vi "Multi-Device_Sync-AI_and_AO-Shared_Timebase_&_Trig-DSA.vi"() -> ()   [LabVIEW 2013]
doc: "I. Description:\nThis example configures a total of four tasks on two PXI Dynamic Signal Acquistion (DSA) devices. Each device runs a task for analog input and another for analog output. This VI illustrates continuous analog input and ouptut operations.\n\nII. Instructions for Running:\n1. Select which type of Syncrhonization method you want to use.\n2. Select the physical channels to corresponding to the signal connection on each device.\n3. Enter the minimum and maximum expected voltage for the input and output operations on each device.\nNote: For optimal accuracy, match the input range to the expected voltage level of the measured signal (for input) and generated signal (for output).\n4. Set the number of samples to acquire per channel. This parameter determines how many points will be read and generated with each iteration of the WHILE loop.\n5. Set the rate of the acquisition and generation. The same sampling rate is employed for input and output operations on each device.\nNote: The sampling rate should be at least 2.2 times the maximum frequency component of the signal being acquired on analog input and the signal being generated on analog output. Frequency components beyond about 0.47 times the sampling rate will be eliminated by the alias and imaging protection on the DSA device.\n\nIII. Block Diagram Steps:\n1. Create an analog input and output channel for both the master and slave devices.\n2. Set timing parameters for a continuous acquisition. The sample rate and block size are set to the same values for each device.\n3. There are two types of synchronization available on DSA devices. The first method shares the Sample Clock Timebase across the PXI_Star bus. It also uses the Sync Pulse which is shared across the PXI_Trig / RTSI bus. The second method uses the Sync Pulse in conjunction with the PXI Reference clock 10 on the PXI backplane. \n4. Call the Get Terminal Name with Device Prefix VI to append the device name to the signal name for the acquisition start trigger. This signal is then used as an output generation trigger on the master as well as and acquisition start trigger and generation start trigger on the slave. The signal is shared along the PXI_Trig / RTSI bus.\n5. Synthesize a standard waveform (sine, square, or triangle) and load this data into the output RAM buffer for each device.\n6. Call the Start VI to start the acquisition and generation tasks. (Note: The flat case structure provides flow control so that the slave device is armed before the master so that the slave device does not miss the trigger.)\n7. Read all of the waveform data from both devices.\n8. Check the status of the analog output tasks on both devices.\n9. Call the Clear Task VI to stop the acquisition and generation and clear the task.\n10. Use the popup dialog box to display an error if any.\n\nIV. I/O Connections Overview:\nMake sure your signal input and output terminals matches the Physical Channel I/O controls.\n\nIt is important to ensure that your PXI chassis has been properly configured in MAX. If your chassis has not been configured in software before running the VI, your devices may fail to synchronize properly."
uses:
  <vilib>/Utility/error.llb/DialogType.ctl
  <vilib>/DAQmx/write.llb/DAQmx Write (Analog Wfm 1Chan NSamp).vi
  <vilib>/DAQmx/read.llb/DAQmx Read (Analog 1D Wfm NChan NSamp).vi
  <vilib>/DAQmx/create/channels.llb/DAQmx Create Channel (AI-Voltage-Basic).vi
  <vilib>/DAQmx/create/channels.llb/DAQmx Create Channel (AO-Voltage-Basic).vi
  <vilib>/DAQmx/configure/timing.llb/DAQmx Timing (Sample Clock).vi
  <vilib>/DAQmx/configure/trigger.llb/DAQmx Start Trigger (Digital Edge).vi
  <vilib>/DAQmx/miscellaneous.llb/DAQmx Fill In Error Info.vi
  <resource>/objmgr/daqmx.rc
panel:
  in  "Synchronization Type":u16(ring) items=["DSA Sample Clock Timebase", "DSA Reference Clock"]
  out "Resulting Sample \nClock Rate [S/s]":dbl format="%.2f"
  in  "Desired Frequency":dbl=1000.0 format="%.2f"
  in  "Cycles per Buffer":dbl=5.0 format="%.2f"
  in  "Waveform Type":T1(ring)
  in  "Samples per Buffer":dbl=250.0
  in  "Amplitude":dbl=1.0 format="%0.2p"
  in  "Minimum Value":dbl=-10.0 caption="Output Minimum Value" format="%0.2f"
  in  "Maximum Value":dbl=10.0 caption="Output Maximum Value" format="%0.2f"
  in  "Physical Channel":tag="PXI1Slot3/ao0" caption="Slave Output Physical Channels"
  in  "Maximum Value":dbl=10.0 caption="Input Maximum Value" format="%0.2f"
  in  "Minimum Value":dbl=-10.0 caption="Input Minimum Value" format="%0.2f"
  in  "Physical Channel":tag="PXI1Slot3/ai0" caption="Slave Input Physical Channel"
  out "Measurement":waveform(dbl)[](graph) caption="Measurement:  Slave Board"
  in  "Samples per Channel":i32=2000 caption="Samples to Read per Loop"
  in  "Minimum Value":dbl=-10.0 caption="Output Minimum Value" format="%0.2f"
  in  "Maximum Value":dbl=10.0 caption="Output Maximum Value" format="%0.2f"
  in  "Physical Channel":tag="PXI1Slot2/ao0" caption="Master Output Physical Channels"
  in  "Maximum Value":dbl=10.0 caption="Input Maximum Value" format="%0.2f"
  in  "Minimum Value":dbl=-10.0 caption="Input Minimum Value" format="%0.2f"
  in  "Physical Channel":tag="PXI1Slot2/ai0" caption="Master Input Physical Channel"
  in  "stop":bool
  out "Measurement":waveform(dbl)[](graph) caption="Measurement:  Master Board"
  # "For instructions, select Help>>Show Context Help"
  # "Channel Parameters:  Master Board"
  # "Channel Parameters:  Slave Board"
  # "Timing Parameters"
  # "Waveform Information"
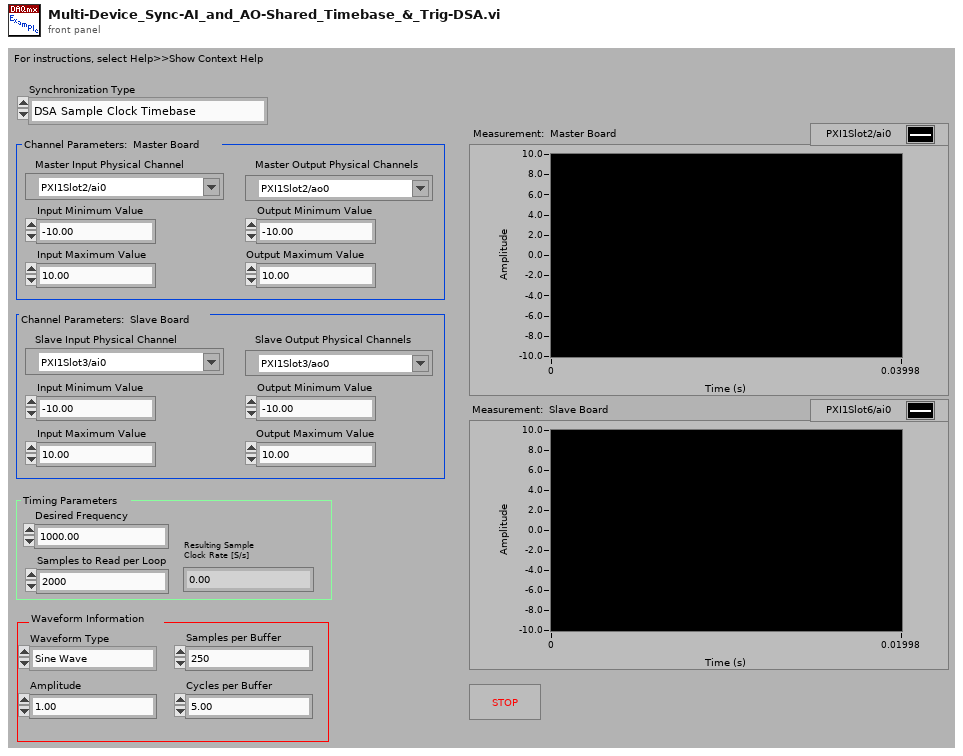
[diagram p1: front panel]
types:
  T1 = enum16{"Sine Wave", "Triangle Wave", "Square Wave", "Sawtooth Wave"}
  T2 = typedef "DialogType.ctl" = u16
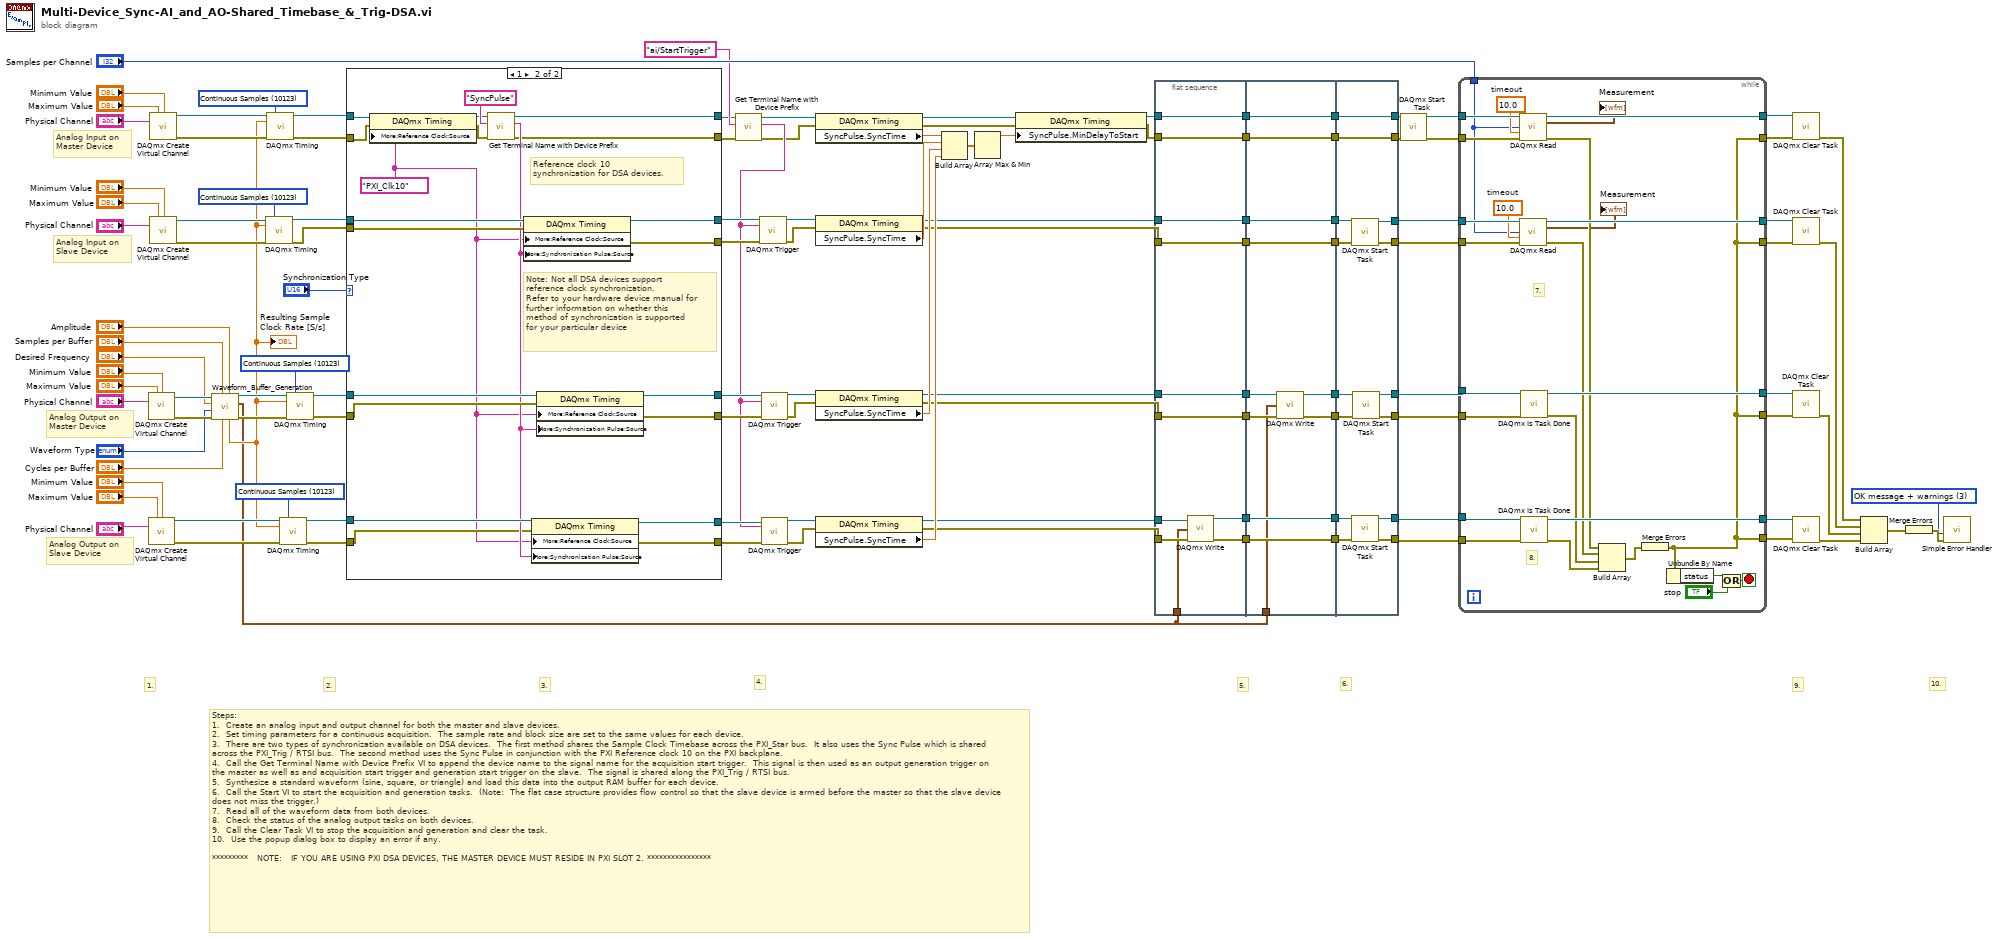
[diagram p0: block diagram]
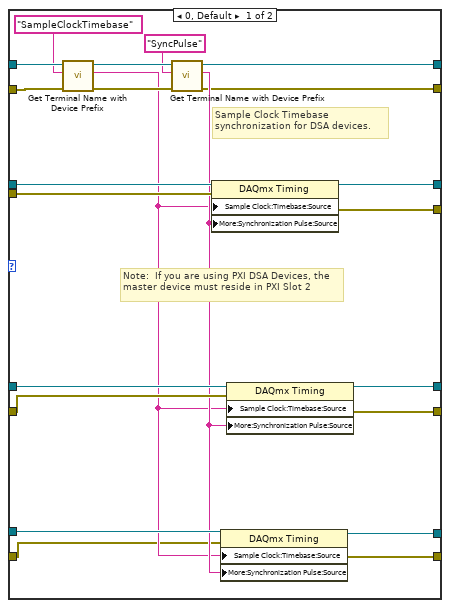
[diagram p2: hidden frame]
diagram:
  w61 = T2 3 items=["no dialog", "OK message", "continue or stop message", "OK message + warnings", "continue/stop + warnings"] ("type of dialog (OK msg:1)")
  w101 = 10123 items=["Finite Samples"=10178, "Continuous Samples"=10123] ("sample mode")
  w102 = 10123 items=["Finite Samples"=10178, "Continuous Samples"=10123] ("sample mode")
  w109 = 10123 items=["Finite Samples"=10178, "Continuous Samples"=10123] ("sample mode")
  w114 = 10123 items=["Finite Samples"=10178, "Continuous Samples"=10123] ("sample mode")
  # "Analog Output on\nMaster Device"
  # "Analog Output on\nSlave Device"
  # "Analog Input on\nSlave Device"
  # "Analog Input on\nMaster Device"
  # "10."
  # "9."
  # "Steps: \n1.  Create an analog input and output channel for both the master and slave devices.\n2.  Set timing parameters for a continuous acquisition.  The sample rate and block size are set to the same values for each device.\n3.  There are two types of synchronization available on DSA devices.  The first method shares the Sample Clock Timebase across the PXI_Star bus.  It also uses the Sync Pulse which is shared across the PXI_Trig / RTSI bus.  The second method uses the Sync Pulse in conjunction with the PXI Reference clock 10 on the PXI backplane. \n4.  Call the Get Terminal Name with Device Prefix VI to append the device name to the signal name for the acquisition start trigger.  This signal is then used as an output generation trigger on the master as well as and acquisition start trigger and generation start trigger on the slave.  The signal is shared along the PXI_Trig / RTSI bus.\n5.  Synthesize a standard waveform (sine, square, or triangle) and load this data into the output RAM buffer for each device.\n6.  Call the Start VI to start the acquisition and generation tasks.  (Note:  The flat case structure provides flow control so that the slave device is armed before the master so that the slave device does not miss the trigger.)\n7.  Read all of the waveform data from both devices.\n8.  Check the status of the analog output tasks on both devices.\n9.  Call the Clear Task VI to stop the acquisition and generation and clear the task.\n10.  Use the popup dialog box to display an error if any.\n\n*********   NOTE:  \tIF YOU ARE USING PXI DSA DEVICES, THE MASTER DEVICE MUST RESIDE IN PXI SLOT 2. ****************"
  # "6."
  # "5."
  # "4."
  # "3."
  # "2."
  # "1."
  n1 = call-poly <vilib>:"DAQmx Create Virtual Channel.vi"("maximum value"="Maximum Value", "minimum value"="Minimum Value", "physical channels"="Physical Channel") -> ("task out"=w68:refnum<k21>, "error out"=w67:errorcluster)  [unwired: 11 in]
  n2 = call-poly <vilib>:"DAQmx Create Virtual Channel.vi"("maximum value"="Maximum Value", "minimum value"="Minimum Value", "physical channels"="Physical Channel") -> ("task out"=w100:refnum<k21>, "error out"=w99:errorcluster)  [unwired: 11 in]
  n3 = call-poly <vilib>:"DAQmx Create Virtual Channel.vi"("maximum value"="Maximum Value", "minimum value"="Minimum Value", "physical channels"="Physical Channel") -> ("task out"=w116:refnum<k21>, "error out"=w118:errorcluster)  [unwired: 11 in]
  n4 = call-poly <vilib>:"DAQmx Create Virtual Channel.vi"("maximum value"="Maximum Value", "minimum value"="Minimum Value", "physical channels"="Physical Channel") -> ("task out"=w111:refnum<k21>, "error out"=w113:errorcluster)  [unwired: 11 in]
  n5 = call "Waveform_Buffer_Generation.vi"("Amplitude"="Amplitude", "Cycles per Buffer"="Cycles per Buffer", "Samples per Buffer"="Samples per Buffer", "error in (no error)"=w67, "Waveform Type"="Waveform Type", "Desired Frequency"="Desired Frequency", "task/channels in"=w68) -> ("error out"=w66:errorcluster, "Waveform"=w1:waveform(dbl), "task out"=w69:refnum<k21>, "Resulting Sample Clock Rate"=w51:dbl)  [unwired: 1 out]
  "Resulting Sample \nClock Rate [S/s]" <- w51
  n6 = call-poly <vilib>:"DAQmx Timing.vi"("task/channels in"=w111, "sample mode"=w109, "rate"=w51, "error in"=w113) -> ("task out"=w106:refnum<k21>, "error out"=w105:errorcluster)  [unwired: 10 in]
  n7 = call-poly <vilib>:"DAQmx Timing.vi"("task/channels in"=w116, "sample mode"=w114, "rate"=w51, "error in"=w118) -> ("task out"=w104:refnum<k21>, "error out"=w103:errorcluster)  [unwired: 10 in]
  n8 = call-poly <vilib>:"DAQmx Timing.vi"("task/channels in"=w100, "sample mode"=w101, "rate"=w51, "error in"=w99) -> ("task out"=w76:refnum<k21>, "error out"=w53:errorcluster)  [unwired: 10 in]
  n9 = call-poly <vilib>:"DAQmx Timing.vi"("task/channels in"=w69, "sample mode"=w102, "rate"=w51, "error in"=w66) -> ("task out"=w60:refnum<k21>, "error out"=w59:errorcluster)  [unwired: 10 in]
  n10 = case shown="1" "Synchronization Type" {
    tunnel: [w140 w161] -> w108
    tunnel: [w139 w160] -> w107
    tunnel: w106 -> [w138 w159]
    tunnel: w105 -> [w137 w158]
    tunnel: w104 -> [w136 w146]
    tunnel: w103 -> [w132 w143]
    tunnel: w76 -> [w130 w156]
    tunnel: [w120 w142] -> w44
    tunnel: [w119 w141] -> w43
    tunnel: w60 -> [w129 w155]
    tunnel: w59 -> [w128 w154]
    tunnel: w53 -> [w125 w152]
    tunnel: [w124 w151] -> w50
    tunnel: [w123 w150] -> w49
    tunnel: [w122 w149] -> w48
    tunnel: [w121 w148] -> w47
    frame 0, Default {
      # "Note:  If you are using PXI DSA Devices, the master device must reside in PXI Slot 2"
      # "Sample Clock Timebase \nsynchronization for DSA devices."
      n11 = call "Get Terminal Name with Device Prefix.vi"("error in (no error)"=w132, "Local Terminal Name"="SampleClockTimebase", "task/channels in"=w136) -> ("error out"=w131:errorcluster, "Terminal Name with Device Prefix"=w126:tag, "task out"=w135:refnum<k21>)  [unwired: 6 in]
      n12 = call "Get Terminal Name with Device Prefix.vi"("error in (no error)"=w131, "Local Terminal Name"="SyncPulse", "task/channels in"=w135) -> ("error out"=w119:errorcluster, "Terminal Name with Device Prefix"=w127:tag, "task out"=w120:refnum<k21>)  [unwired: 6 in]
      n13 = property class="DAQmx Timing"(reference=w138, error in=w137, "Sample Clock:Timebase:Source"=w126, "More:Synchronization Pulse:Source"=w127) -> (reference out=w140:refnum<k21>, error out=w139:errorcluster)
      n14 = property class="DAQmx Timing"(reference=w130, error in=w125, "Sample Clock:Timebase:Source"=w126, "More:Synchronization Pulse:Source"=w127) -> (reference out=w122:refnum<k21>, error out=w121:errorcluster)
      n15 = property class="DAQmx Timing"(reference=w129, error in=w128, "Sample Clock:Timebase:Source"=w126, "More:Synchronization Pulse:Source"=w127) -> (reference out=w124:refnum<k21>, error out=w123:errorcluster)
    }
    frame 1 {
      w145 = tag "PXI_Clk10" ("RefClk.Src")
      # "Note: Not all DSA devices support\nreference clock synchronization.\nRefer to your hardware device manual for\nfurther information on whether this \nmethod of synchronization is supported\nfor your particular device"
      # "Reference clock 10\nsynchronization for DSA devices."
      n16 = property class="DAQmx Timing"(reference=w146, error in=w143, "More:Reference Clock:Source"=w145) -> (reference out=w147:refnum<k21>, error out=w144:errorcluster)
      n17 = call "Get Terminal Name with Device Prefix.vi"("error in (no error)"=w144, "Local Terminal Name"="SyncPulse", "task/channels in"=w147) -> ("error out"=w141:errorcluster, "Terminal Name with Device Prefix"=w153:tag, "task out"=w142:refnum<k21>)  [unwired: 6 in]
      n18 = property class="DAQmx Timing"(reference=w159, error in=w158, "More:Reference Clock:Source"=w145, "More:Synchronization Pulse:Source"=w153) -> (reference out=w161:refnum<k21>, error out=w160:errorcluster)
      n19 = property class="DAQmx Timing"(reference=w156, error in=w152, "More:Reference Clock:Source"=w145, "More:Synchronization Pulse:Source"=w153) -> (reference out=w149:refnum<k21>, error out=w148:errorcluster)
      n20 = property class="DAQmx Timing"(reference=w155, error in=w154, "More:Reference Clock:Source"=w145, "More:Synchronization Pulse:Source"=w153) -> (reference out=w151:refnum<k21>, error out=w150:errorcluster)
    }
  }
  n21 = call "Get Terminal Name with Device Prefix.vi"("error in (no error)"=w43, "Local Terminal Name"="ai/StartTrigger", "task/channels in"=w44) -> ("error out"=w40:errorcluster, "Terminal Name with Device Prefix"=w42:tag, "task out"=w41:refnum<k21>)  [unwired: 6 in]
  n22 = call-poly <vilib>:"DAQmx Trigger.vi"("task/channels in"=w108, "source"=w42, "error in"=w107) -> ("task out"=w36:refnum<k21>, "error out"=w37:errorcluster)  [unwired: 11 in]
  n23 = call-poly <vilib>:"DAQmx Trigger.vi"("task/channels in"=w50, "source"=w42, "error in"=w49) -> ("task out"=w34:refnum<k21>, "error out"=w35:errorcluster)  [unwired: 11 in]
  n24 = call-poly <vilib>:"DAQmx Trigger.vi"("task/channels in"=w48, "source"=w42, "error in"=w47) -> ("task out"=w39:refnum<k21>, "error out"=w38:errorcluster)  [unwired: 11 in]
  n25 = property class="DAQmx Timing"(reference=w41, error in=w40) -> (reference out=w31:refnum<k21>, error out=w32:errorcluster, "SyncPulse.SyncTime"=w33:dbl)
  n26 = property class="DAQmx Timing"(reference=w36, error in=w37) -> (reference out=w22:refnum<k21>, error out=w23:errorcluster, "SyncPulse.SyncTime"=w28:dbl)
  n27 = property class="DAQmx Timing"(reference=w34, error in=w35) -> (reference out=w10:refnum<k21>, error out=w12:errorcluster, "SyncPulse.SyncTime"=w27:dbl)
  n28 = property class="DAQmx Timing"(reference=w39, error in=w38) -> (reference out=w8:refnum<k21>, error out=w9:errorcluster, "SyncPulse.SyncTime"=w26:dbl)
  n29 = Build Array(w33, w28, w27, w26) -> (w30:dbl[])
  n30 = Array Max & Min(array=w30) -> (max value=w29:dbl)  [unwired: 3 out]
  n31 = property class="DAQmx Timing"(reference=w31, error in=w32, "SyncPulse.MinDelayToStart"=w29) -> (reference out=w24:refnum<k21>, error out=w25:errorcluster)
  n32 = flat-sequence {
    tunnel: w25 -> [w169]
    tunnel: w24 -> [w170]
    tunnel: w23 -> [w171]
    tunnel: w22 -> [w172]
    tunnel: [w172] -> w17
    tunnel: [w171] -> w16
    tunnel: [w170] -> w15
    tunnel: [w169] -> w14
    tunnel: [w168] -> w13
    tunnel: w12 -> [w168]
    tunnel: [w167] -> w11
    tunnel: w10 -> [w167]
    tunnel: w9 -> [w166]
    tunnel: w8 -> [w165]
    tunnel: [w164] -> w6
    tunnel: [w163] -> w4
    tunnel: w1 -> [w162]
    tunnel: [w183] -> w21
    tunnel: [w182] -> w20
    tunnel: [w181] -> w19
    tunnel: [w180] -> w18
    tunnel: w17 -> [w183]
    tunnel: w16 -> [w182]
    tunnel: w15 -> [w181]
    tunnel: w14 -> [w180]
    tunnel: w13 -> [w179]
    tunnel: w11 -> [w178]
    tunnel: [w177] -> w7
    tunnel: w6 -> [w177]
    tunnel: [w176] -> w5
    tunnel: w4 -> [w176]
    tunnel: [w175] -> w3
    tunnel: [w174] -> w2
    tunnel: w1 -> [w173]
    tunnel: [w190] -> w72
    tunnel: [w191] -> w73
    tunnel: [w192] -> w70
    tunnel: [w193] -> w71
    tunnel: [w194] -> w74
    tunnel: [w196] -> w75
    tunnel: [w189] -> w58
    tunnel: [w188] -> w56
    tunnel: w21 -> [w197]
    tunnel: w20 -> [w195]
    tunnel: w19 -> [w189]
    tunnel: w18 -> [w188]
    tunnel: w7 -> [w187]
    tunnel: w5 -> [w186]
    tunnel: w3 -> [w185]
    tunnel: w2 -> [w184]
    frame #0 {
      n33 = call-poly <vilib>:"DAQmx Write.vi"("task/channels in"=w165, "data"=w162, "error in"=w166) -> ("task out"=w163:refnum<k21>, "error out"=w164:errorcluster)  [unwired: 10 in, 1 out]
    }
    frame #1 {
      n34 = call-poly <vilib>:"DAQmx Write.vi"("task/channels in"=w178, "data"=w173, "error in"=w179) -> ("task out"=w174:refnum<k21>, "error out"=w175:errorcluster)  [unwired: 10 in, 1 out]
    }
    frame #2 {
      n35 = call <vilib>:"DAQmx Start Task.vi"("task/channels in"=w197, "error in"=w195) -> ("task out"=w196:refnum<k21>, "error out"=w194:errorcluster)  [unwired: 12 in]
      n36 = call <vilib>:"DAQmx Start Task.vi"("task/channels in"=w186, "error in"=w187) -> ("task out"=w193:refnum<k21>, "error out"=w192:errorcluster)  [unwired: 12 in]
      n37 = call <vilib>:"DAQmx Start Task.vi"("task/channels in"=w184, "error in"=w185) -> ("task out"=w191:refnum<k21>, "error out"=w190:errorcluster)  [unwired: 12 in]
    }
  }
  n38 = call <vilib>:"DAQmx Start Task.vi"("task/channels in"=w58, "error in"=w56) -> ("task out"=w57:refnum<k21>, "error out"=w55:errorcluster)  [unwired: 12 in]
  n39 = while {
    tunnel: [w204] -> w117
    tunnel: w57 -> [w223]
    tunnel: [w222] -> w115
    tunnel: [w204] -> w112
    tunnel: w75 -> [w220]
    tunnel: [w219] -> w110
    tunnel: w73 -> [w217]
    tunnel: w71 -> [w216]
    tunnel: w55 -> [w207]
    tunnel: [w215] -> w98
    tunnel: [w214] -> w97
    tunnel: [w204] -> w96
    tunnel: [w204] -> w95
    tunnel: w74 -> [w208]
    tunnel: w70 -> [w206]
    tunnel: w72 -> [w205]
    tunnel: "Samples per Channel" -> [w203]
    stop <- w211 stop-if-true
    w218 = 10.0  # timeout
    w221 = 10.0  # timeout
    # "8."
    # "7."
    n40 = call-poly <vilib>:"DAQmx Read.vi"("task/channels in"=w223, "number of samples per channel"=w203, "timeout"=w221, "error in"=w207) -> ("task out"=w222:refnum<k21>, "data"=→"Measurement":waveform(dbl)[], "error out"=w200:errorcluster)  [unwired: 9 in]
    n41 = call-poly <vilib>:"DAQmx Read.vi"("task/channels in"=w220, "number of samples per channel"=w203, "timeout"=w218, "error in"=w208) -> ("task out"=w219:refnum<k21>, "data"=→"Measurement":waveform(dbl)[], "error out"=w201:errorcluster)  [unwired: 9 in]
    n42 = call <vilib>:"DAQmx Is Task Done.vi"("task/channels in"=w217, "error in"=w205) -> ("task out"=w215:refnum<k21>, "error out"=w202:errorcluster)  [unwired: 11 in, 1 out]
    n43 = call <vilib>:"DAQmx Is Task Done.vi"("task/channels in"=w216, "error in"=w206) -> ("task out"=w214:refnum<k21>, "error out"=w210:errorcluster)  [unwired: 11 in, 1 out]
    n44 = Build Array(w200, w201, w202, w210) -> (w213:errorcluster[])
    n45 = Merge Errors(w213) -> (w204:errorcluster)
    n46 = Unbundle By Name(w204) -> ("status"=w212:bool)
    n47 = Or(x=w212, y="stop") -> (x .or. y?=w211:bool)
  }
  n48 = call <vilib>:"DAQmx Clear Task.vi"("task in"=w115, "error in"=w117) -> ("error out"=w94:errorcluster)  [unwired: 13 in]
  n49 = call <vilib>:"DAQmx Clear Task.vi"("task in"=w110, "error in"=w112) -> ("error out"=w93:errorcluster)  [unwired: 13 in]
  n50 = call <vilib>:"DAQmx Clear Task.vi"("task in"=w98, "error in"=w96) -> ("error out"=w92:errorcluster)  [unwired: 13 in]
  n51 = call <vilib>:"DAQmx Clear Task.vi"("task in"=w97, "error in"=w95) -> ("error out"=w91:errorcluster)  [unwired: 13 in]
  n52 = Build Array(w94, w93, w92, w91) -> (w90:errorcluster[])
  n53 = Merge Errors(w90) -> (w89:errorcluster)
  n54 = call <vilib>:"Simple Error Handler.vi"("type of dialog (OK msg:1)"=w61, "error in (no error)"=w89) -> ()  [unwired: 3 in, 5 out]
